vi "Open.vi"(4 "Max Value":dbl[](array[numeric]), 6 "Min Value":dbl[](array[numeric]), 7 "Allow multiple opens?":bool, 8 "error in (no error)":errorcluster, 10 "Channel Names":tag[](array[tag])) -> (0 "error out":errorcluster, 3 "AI (N Samples) Ref Out":T1)   [LabVIEW 2021, in "AI Block.lvlib"]
doc: "Opens a reference to analog input block read channel (Connector A/AI0). You must open a reference before you read values from the analog input block read channel."
uses:
  <vilib>/myRIO/Instrument Drivers/Onboard IO/AI Block/AI Block.lvlib
  <vilib>/myRIO/Instrument Drivers/Onboard IO/AI Block/typedefs/AI Block Reference.ctl
  <vilib>/myRIO/Common/Instrument Driver Framework/Utilities/typedefs/myRIO Generic Hardware Reference.ctl
  <vilib>/myRIO/Common/Instrument Driver Framework/Utilities/typedefs/Hardware Version Enum.ctl
  <vilib>/myRIO/Common/Instrument Driver Framework/Utilities/typedefs/myRIO v1.0 Reference.ctl
  <vilib>/myRIO/Common/Instrument Driver Framework/Utilities/typedefs/Generic FPGA Reference.ctl
  <vilib>/myRIO/Common/Instrument Driver Framework/myRIO v1.0/AI Block/typedefs/AI Block Channels List.ctl
  <vilib>/myRIO/Common/Instrument Driver Framework/myRIO v1.0/AI Block/typedefs/AI Block Channels Enum.ctl
  <vilib>/myRIO/Common/Instrument Driver Framework/Utilities/typedefs/Analog Scaling Constants.ctl
  <vilib>/userdefined/High Color/nirio_resource_hc.ctl
panel:
  # "AI (N Samples) Open"
  # "Opens a reference to the myRIO hardware and configures the AI (N Samples) Reference with channels to be read"
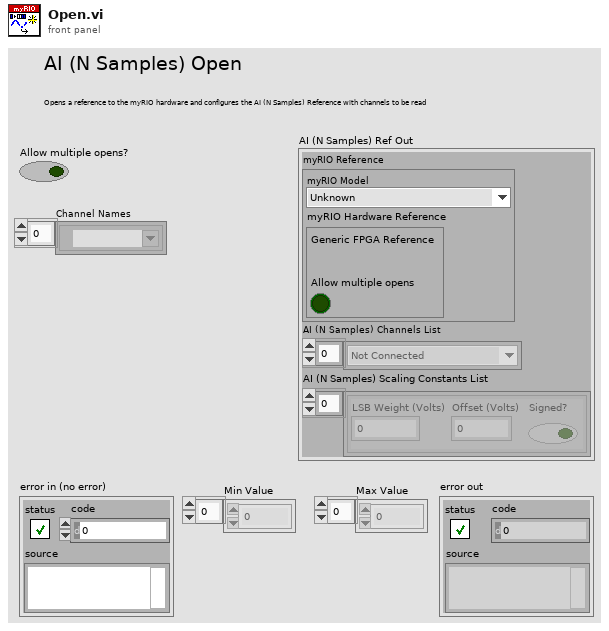
[diagram p1: front panel]
types:
  T1 = typedef "AI Block.lvlib/AI Block Reference.ctl" = cluster{"myRIO Reference":T2, "AI (N Samples) Channels List":T6, "AI (N Samples) Scaling Constants List":T8[]}
  T2 = typedef "myRIO Generic Hardware Reference.ctl" = cluster{"myRIO Model":T3, "myRIO Hardware Reference":T4}
  T3 = typedef "Hardware Version Enum.ctl" = enum16{"Unknown", "myRIO-1900", "myRIO-1950", "roboRIO", "NI ELVIS RIO CM", "ELVIS III"}
  T4 = typedef "myRIO v1.0 Reference.ctl" = cluster{"Generic FPGA Reference":T5, "Allow multiple opens":bool}
  T5 = typedef "Generic FPGA Reference.ctl" = refnum<k20>
  T6 = typedef "AI Block Channels List.ctl" = T7[]
  T7 = typedef "AI Block Channels Enum.ctl" = enum16{"Not Connected", "A/AI0 (N Samples)", "A/AI1 (N Samples)", "A/AI2 (N Samples)", "A/AI3 (N Samples)", "A/AI4 (N Samples)", "A/AI5 (N Samples)", "A/AI6 (N Samples)", "A/AI7 (N Samples)", "A/AI0 (DIFF N Samples)", "A/AI1 (DIFF N Samples)", "A/AI2 (DIFF N Samples)", "A/AI3 (DIFF N Samples)", "B/AI0 (N Samples)", "B/AI1 (N Samples)", "B/AI2 (N Samples)", "B/AI3 (N Samples)", "B/AI4 (N Samples)", "B/AI5 (N Samples)", "B/AI6 (N Samples)", "B/AI7 (N Samples)", "B/AI0 (DIFF N Samples)", "B/AI1 (DIFF N Samples)", "B/AI2 (DIFF N Samples)", "B/AI3 (DIFF N Samples)"}
  T8 = typedef "Analog Scaling Constants.ctl" = cluster{"LSB Weight (Volts)":dbl, "Offset (Volts)":dbl, "Signed?":bool}
  T9 = typedef "nirio_resource_hc.ctl" = tag
  T10 = typedef "Analog Scaling Constants List.ctl" = T8[]
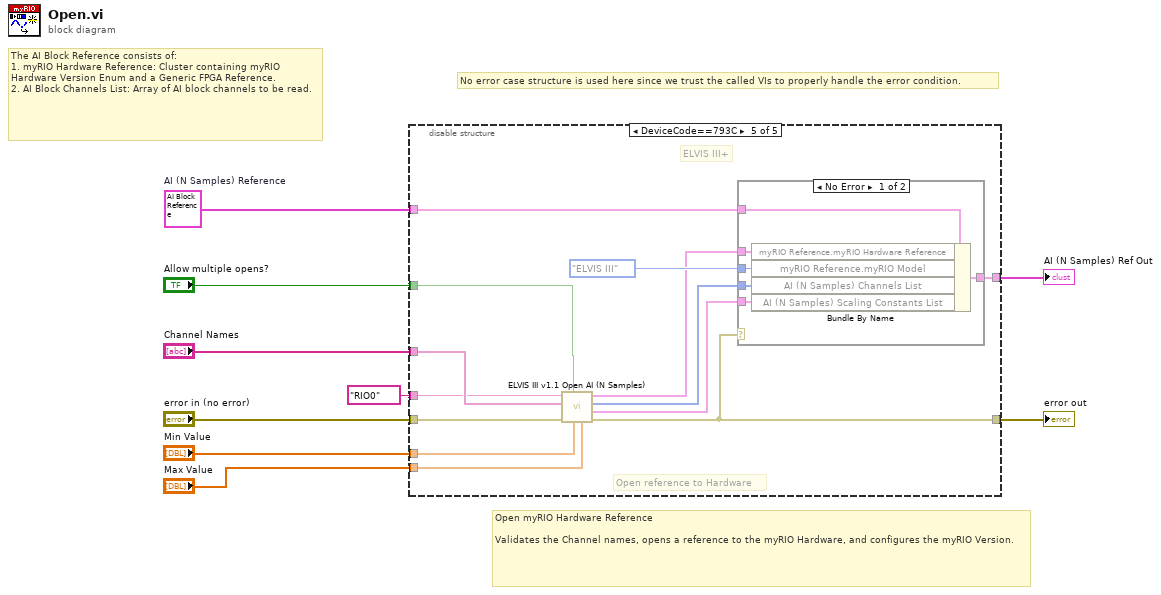
[diagram p0: block diagram]
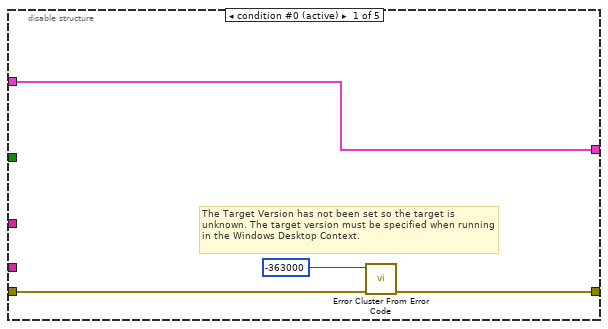
[diagram p2: hidden frame]
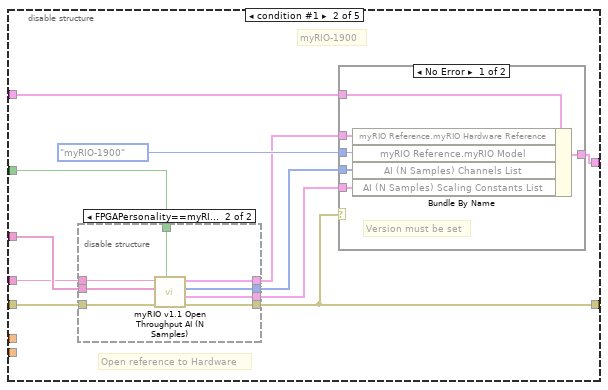
[diagram p3: hidden frame]
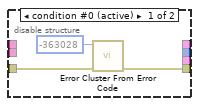
[diagram p4: hidden frame]
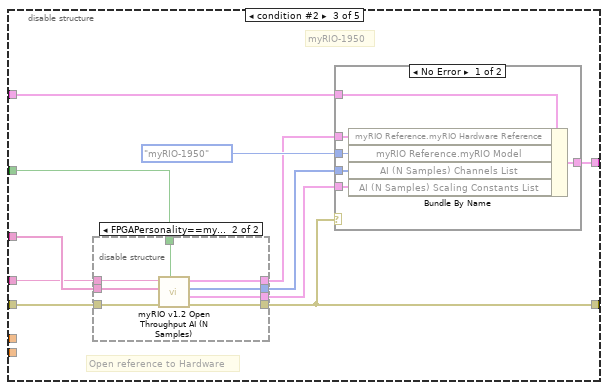
[diagram p6: hidden frame]
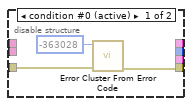
[diagram p7: hidden frame]
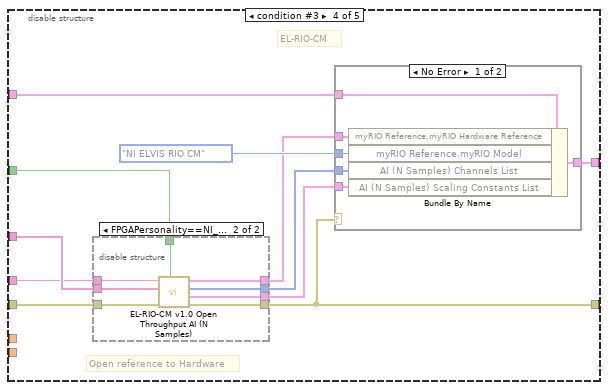
[diagram p9: hidden frame]
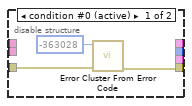
[diagram p10: hidden frame]
diagram:
  w4 = T1 {"myRIO Reference"={"myRIO Model"=enum."Unknown", "myRIO Hardware Reference"={"Generic FPGA Reference"=refnum, "Allow multiple opens"=FALSE}}, "AI (N Samples) Channels List"=[], "AI (N Samples) Scaling Constants List"=[]}  # AI (N Samples) Reference
  # "No error case structure is used here since we trust the called VIs to properly handle the error condition."
  # "The AI Block Reference consists of:\n1. myRIO Hardware Reference: Cluster containing myRIO Hardware Version Enum and a Generic FPGA Reference.\n2. AI Block Channels List: Array of AI block channels to be read."
  # "Open myRIO Hardware Reference\n\nValidates the Channel names, opens a reference to the myRIO Hardware, and configures the myRIO Version."
  n1 = disable-structure shown="DeviceCode==793C" {
    disable-tunnel: [w13 w16 w45 w74 w101] -> w6
    disable-tunnel: "Channel Names" -> [_ w24 w53 w82 w107]
    disable-tunnel: "Allow multiple opens?" -> [_ w20 w52 w81 w108]
    disable-tunnel: [w10 w23 w51 w80 w102] -> w5
    disable-tunnel: "error in (no error)" -> [w12 w21 w49 w78 w105]
    disable-tunnel: w4 -> [w10 w19 w47 w76 w109]
    disable-tunnel: T9 "RIO0" ("Resource name") -> [_ w17 w46 w75 w106]
    disable-tunnel: "Min Value" -> [_ _ _ _ w104]
    disable-tunnel: "Max Value" -> [_ _ _ _ w103]
    frame condition #0 (active) {
      # "The Target Version has not been set so the target is unknown. The target version must be specified when running in the Windows Desktop Context."
      n2 = call <vilib>:"Error Cluster From Error Code.vi"("error in (no error)"=w12, "error code (0)"=-363000) -> ("error out"=w13:errorcluster)  [unwired: 7 in]
    }
    frame condition #1 {
      # "myRIO-1900"
      # "Open reference to Hardware"
      n3 = disable-structure shown="FPGAPersonality==myRIO_FP_Throughput" {
        disable-tunnel: w24 -> [_ w33]
        disable-tunnel: w21 -> [w26 w32]
        disable-tunnel: w20 -> [_ w35]
        disable-tunnel: [_ w30] -> w18
        disable-tunnel: w17 -> [_ w34]
        disable-tunnel: [w25 w28] -> w16
        disable-tunnel: [_ w31] -> w15
        disable-tunnel: [_ w29] -> w14
        frame condition #0 (active) {
          n4 = call <vilib>:"Error Cluster From Error Code.vi"("error in (no error)"=w26, "error code (0)"=-363028) -> ("error out"=w25:errorcluster)  [unwired: 7 in]
        }
        frame condition #1 {
          n5 = call <vilib>:"myRIO v1.1 Open Throughput AI (N Samples).vi"("Allow multiple opens?"=w35, "error in (no error)"=w32, "Channel Names"=w33, "Resource name"=w34) -> ("error out"=w28:errorcluster, "AI (N Samples) Scale Constants List"=w29:T10, "AI (N Samples) Channel List"=w30:T6, "myRIO Ref Out"=w31:T4)  [unwired: 4 in]
        }
      }
      n6 = case shown="No Error" w16 {
        tunnel: [w41 w42] -> w23
        tunnel: Hardware_Version_Enum."myRIO-1900" ("Hardware Version Enum") -> [w40 _]
        tunnel: w19 -> [w39 w42]
        tunnel: w18 -> [w37 _]
        tunnel: w15 -> [w38 _]
        tunnel: w14 -> [w36 _]
        frame No Error {
          # "Version must be set"
          n7 = Bundle By Name(cluster=w39, "myRIO Reference.myRIO Hardware Reference"=w38, "myRIO Reference.myRIO Model"=w40, "AI (N Samples) Channels List"=w37, "AI (N Samples) Scaling Constants List"=w36) -> (w41:T1)
        }
        frame Error {
        }
      }
    }
    frame condition #2 {
      # "myRIO-1950"
      # "Open reference to Hardware"
      n8 = disable-structure shown="FPGAPersonality==myRIO_FP_Throughput" {
        disable-tunnel: w53 -> [_ w62]
        disable-tunnel: w52 -> [_ w64]
        disable-tunnel: w49 -> [w55 w61]
        disable-tunnel: [_ w60] -> w48
        disable-tunnel: w46 -> [_ w63]
        disable-tunnel: [w54 w57] -> w45
        disable-tunnel: [_ w59] -> w44
        disable-tunnel: [_ w58] -> w43
        frame condition #0 (active) {
          n9 = call <vilib>:"Error Cluster From Error Code.vi"("error in (no error)"=w55, "error code (0)"=-363028) -> ("error out"=w54:errorcluster)  [unwired: 7 in]
        }
        frame condition #1 {
          n10 = call <vilib>:"myRIO v1.2 Open Throughput AI (N Samples).vi"("Allow multiple opens?"=w64, "error in (no error)"=w61, "Channel Names"=w62, "Resource name"=w63) -> ("error out"=w57:errorcluster, "AI (N Samples) Scale Constants List"=w58:T10, "AI (N Samples) Channel List"=w59:T6, "myRIO Ref Out"=w60:T4)  [unwired: 4 in]
        }
      }
      n11 = case shown="No Error" w45 {
        tunnel: [w70 w71] -> w51
        tunnel: Hardware_Version_Enum."myRIO-1950" ("Hardware Version Enum") -> [w69 _]
        tunnel: w48 -> [w66 _]
        tunnel: w47 -> [w68 w71]
        tunnel: w44 -> [w67 _]
        tunnel: w43 -> [w65 _]
        frame No Error {
          n12 = Bundle By Name(cluster=w68, "myRIO Reference.myRIO Hardware Reference"=w66, "myRIO Reference.myRIO Model"=w69, "AI (N Samples) Channels List"=w67, "AI (N Samples) Scaling Constants List"=w65) -> (w70:T1)
        }
        frame Error {
        }
      }
    }
    frame condition #3 {
      # "EL-RIO-CM"
      # "Open reference to Hardware"
      n13 = disable-structure shown="FPGAPersonality==NI_ELVIS_RIO_CM_FP_Throughput" {
        disable-tunnel: w82 -> [_ w91]
        disable-tunnel: w81 -> [_ w93]
        disable-tunnel: w78 -> [w84 w90]
        disable-tunnel: [_ w89] -> w77
        disable-tunnel: w75 -> [_ w92]
        disable-tunnel: [w83 w86] -> w74
        disable-tunnel: [_ w88] -> w73
        disable-tunnel: [_ w87] -> w72
        frame condition #0 (active) {
          n14 = call <vilib>:"Error Cluster From Error Code.vi"("error in (no error)"=w84, "error code (0)"=-363028) -> ("error out"=w83:errorcluster)  [unwired: 7 in]
        }
        frame condition #1 {
          n15 = call <vilib>:"EL-RIO-CM v1.0 Open Throughput AI (N Samples).vi"("Allow multiple opens?"=w93, "error in (no error)"=w90, "Channel Names"=w91, "Resource name"=w92) -> ("error out"=w86:errorcluster, "AI (N Samples) Scale Constants List"=w87:T10, "AI (N Samples) Channel List"=w88:T6, "myRIO Ref Out"=w89:T4)  [unwired: 4 in]
        }
      }
      n16 = case shown="No Error" w74 {
        tunnel: [w99 w100] -> w80
        tunnel: Hardware_Version_Enum."NI ELVIS RIO CM" ("Hardware Version Enum") -> [w98 _]
        tunnel: w77 -> [w95 _]
        tunnel: w76 -> [w97 w100]
        tunnel: w73 -> [w96 _]
        tunnel: w72 -> [w94 _]
        frame No Error {
          n17 = Bundle By Name(cluster=w97, "myRIO Reference.myRIO Hardware Reference"=w95, "myRIO Reference.myRIO Model"=w98, "AI (N Samples) Channels List"=w96, "AI (N Samples) Scaling Constants List"=w94) -> (w99:T1)
        }
        frame Error {
        }
      }
    }
    frame condition #4 {
      # "ELVIS III+"
      # "Open reference to Hardware"
      n18 = call <vilib>:"ELVIS III v1.1 Open AI (N Samples).vi"("Max Value"=w103, "Min Value"=w104, "Allow multiple opens?"=w108, "error in (no error)"=w105, "Channel Names"=w107, "Resource name"=w106) -> ("error out"=w101:errorcluster, "AI (N Samples) Scale Constants List"=w110:T10, "AI (N Samples) Channel List"=w111:T6, "myRIO Ref Out"=w112:T4)  [unwired: 2 in]
      n19 = case shown="No Error" w101 {
        tunnel: [w119 w120] -> w102
        tunnel: Hardware_Version_Enum."ELVIS III" ("Hardware Version Enum") -> [w118 _]
        tunnel: w112 -> [w115 _]
        tunnel: w109 -> [w117 w120]
        tunnel: w111 -> [w116 _]
        tunnel: w110 -> [w114 _]
        frame No Error {
          n20 = Bundle By Name(cluster=w117, "myRIO Reference.myRIO Hardware Reference"=w115, "myRIO Reference.myRIO Model"=w118, "AI (N Samples) Channels List"=w116, "AI (N Samples) Scaling Constants List"=w114) -> (w119:T1)
        }
        frame Error {
        }
      }
    }
  }
  "AI (N Samples) Ref Out" <- w5
  "error out" <- w6
